vi "Create File with New Extension.vi"(5 "Suffix":string, 6 "New File Extension":string, 7 "Prefix":string, 8 "Error In":errorcluster, 9 "Dialog?":bool, 11 "File Path in":path) -> (0 "Error Out":errorcluster, 3 "New File Path out":path)   [LabVIEW 2021, in "Files.lvlib"]
doc: "Takes a file with extension 1 (e.g. <B>.ext</B>) or folder and a new extension 2 (e.g. <B>.tx</B>) and creates a new file with the second extension.\n\nIf a file with that name already exists, adds a number in parenthesis to the name to avoid overwriting the existing file.\n\nNote: if the second extension does not contain a dot, it is added."
uses:
  Files.lvlib
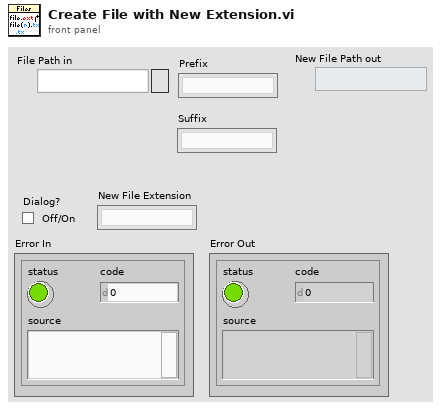
[diagram p1: front panel]
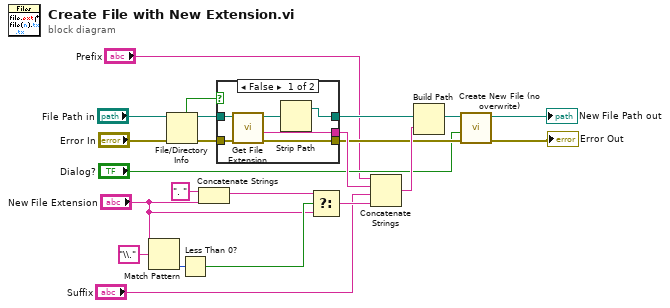
[diagram p0: block diagram]
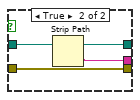
[diagram p2: hidden frame]
diagram:
  n1 = Match Pattern(string="New File Extension", regular expression="\\.") -> (offset past match=w16:i32)  [unwired: 1 in, 3 out]
  n2 = File/Directory Info(path="File Path in", error in="Error In") -> (path out=w7:path, directory=w6:bool, error out=w8:errorcluster)  [unwired: 4 out]
  n3 = Less Than 0?(x=w16) -> (x < 0?=w15:bool)
  n4 = Concatenate Strings(". " ("string"), "New File Extension") -> (w12:string)
  n5 = case shown="False" w6 {
    tunnel: [w23 w29] -> w22
    tunnel: [w27 w30] -> w21
    tunnel: [w26 w31] -> w19
    tunnel: w8 -> [w25 w31]
    tunnel: w7 -> [w24 w32]
    frame False {
      n6 = call <vilib>:"Get File Extension.vi"("error in (no error)"=w25, "file"=w24) -> ("error out"=w26:errorcluster, "filename without extension"=w27:string, "dup file"=w28:path)  [unwired: 5 in, 2 out]
      n7 = Strip Path(path=w28) -> (stripped path=w23:path)  [unwired: 1 out]
    }
    frame True {
      n8 = Strip Path(path=w32) -> (stripped path=w29:path, name=w30:string)
    }
  }
  n9 = Select(t=w12, s=w15, f="New File Extension") -> (s? t:f=w11:string)
  n10 = Concatenate Strings("Prefix", w21, "Suffix", w11) -> (w20:string)
  n11 = Build Path(base path=w22, name or relative path=w20) -> (appended path=w5:path)
  n12 = call "Create New File (no overwrite).vi"("Error In"=w19, "Dialog?"="Dialog?", "New Path"=w5) -> ("Error Out"=→"Error Out":errorcluster, "New (modified) Path"=→"New File Path out":path)  [unwired: 7 in]
